vi "PCSLauncher.read DB.vi"(0 "i ref in":refnum<vi>, 5 "error in (no error)":errorcluster) -> (11 "Captions":T2, 13 "Indicator DIM Service Names":T1, 14 "i ref out":refnum<vi>, 15 "DSC Int Proc":string, 16 "DIM Service Name Select Direction":string, 17 "DIM Service Name Move":string, 18 "PSDB Instance Information: Subsystem":string, 19 "error out":errorcluster)   [LabVIEW 2014]
doc: "This VI reads the data base and stores the information to own attributes."
uses:
  CSCore/BaseProcess/BaseProcess.lvlib
panel:
  in  "Dummy Indicator DIM Service Names":T1
  in  "Captions Dummy":T2
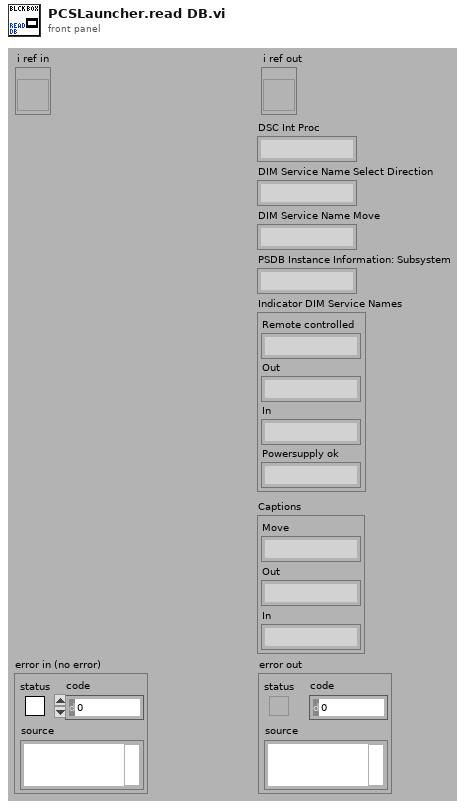
[diagram p1: front panel]
types:
  T1 = cluster{"Remote controlled":string, "Out":string, "In":string, "Powersupply ok":string}
  T2 = cluster{"Move":string, "Out":string, "In":string}
  T3 = typedef "BaseProcess.lvlib/BaseProcess.i attribute.ctl" = cluster{"EventStatus":string, "EventError":i32, "PresetEvtWatchD":i32, "PresetPdcWatchD":i32, "EventTimeout":i32, "PeriodicInterval":i32, "Interface":string[], "Address":string[], "Special":string[], "PeriodicError":i32, "PeriodicStatus":string, "SuperProc":string, "Descriptors":T4[], "CaseRef":refnum<vi>, "PdcRef":refnum<vi>, "Thread Ref":refnum<vi>, "eventErrorID":i32, "eventStatusID":i32, "periodicErrorID":i32, "periodicStatusID":i32, "pdcCtrID":i32}
  T4 = typedef "BaseProcess.lvlib/BaseProcess.descriptor definition.ctl" = cluster{"selector":string, "descriptor":T5}
  T5 = typedef "BaseProcess.lvlib/BaseProcess.descriptor string definition.ctl" = string
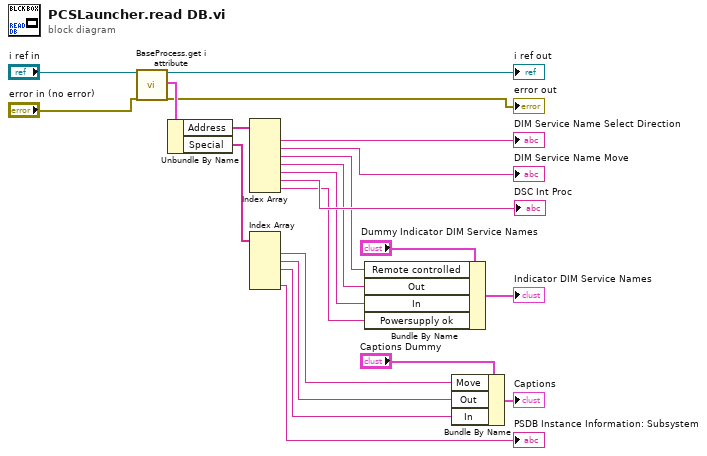
[diagram p0: block diagram]
diagram:
  n1 = call "BaseProcess.get i attribute.vi"("i ref in"="i ref in", "error in (no error)"="error in (no error)") -> ("i ref out"=→"i ref out":refnum<vi>, "i attribute"=w22:T3, "error out"=→"error out":errorcluster)  [unwired: 15 in]
  n2 = Unbundle By Name(w22) -> ("Address"=w21:string[], "Special"=w20:string[])
  n3 = Index Array(array=w21) -> (element #1=→"DIM Service Name Select Direction":string, element #2=→"DIM Service Name Move":string, element #3=w3:string, element #4=w4:string, element #5=w5:string, element #6=→"DSC Int Proc":string, element #7=w6:string)  [unwired: 7 in]
  n4 = Index Array(array=w20) -> (element #1=w13:string, element #2=w12:string, element #3=w11:string, element #5=→"PSDB Instance Information: Subsystem":string)  [unwired: 5 in, 1 out]
  n5 = Bundle By Name(cluster="Dummy Indicator DIM Service Names", "Remote controlled"=w3, "Out"=w4, "In"=w5, "Powersupply ok"=w6) -> (→"Indicator DIM Service Names":T1)
  n6 = Bundle By Name(cluster="Captions Dummy", "Move"=w13, "Out"=w12, "In"=w11) -> (→"Captions":T2)
